vi "Hardware Discovery.vi"() -> ()   [LabVIEW 2020]
uses:
  support/Controls/State Data.ctl
  support/Controls/Targets Settings.ctl
  support/Controls/Target Information.ctl
  support/Controls/Target Network Settings.ctl
  support/Controls/System Credentials.ctl
  support/Controls/Important Paths.ctl
  support/Controls/Exit Button.ctl
  support/Controls/Refresh Button.ctl
  support/Controls/Configure Button.ctl
  support/Controls/Select All Button.ctl
  support/Controls/Add Target Button.ctl
  support/Controls/SetUp Btn.ctl
  support/Controls/FP Control Functions.ctl
  <vilib>/Utility/miscctls.llb/LVRowAndColumnUnsignedTypeDef.ctl
  support/Message Queue/Enqueue Message (Single).vi
  <vilib>/nisyscfg/Close (System).vi
  support/Message Queue/Message Queue.lvlib
  <vilib>/nisyscfg/nisyscfg.lvlib
  <resource>/objmgr/nisysapi.rc
  support/User Event - Stop/User Event - Stop.lvlib
panel:
  in  "App Images List":i32(listbox)=6
  in  "Target List 2":i32[](listbox)=[0]
  out "LinuxRT Version to be applied":string
  in  "Set Up Target":T1
  in  "Exit":T2
  in  "Target List":i32[](listbox)=[0]
  in  "Refresh Targets":T3
  in  "Targets Settings":bool
  in  "Add Target":T4
  in  "Select All":T5
  in  "Configure Targets":T6
  in  "App Data":T7 {"Targets Information"."Primary NIC"."IP Address Request Mode" items=["Static"=1, "DHCP/Link-Local"=2, "Link-Local Only"=4, "DHCP Only"=8]}
  # "Detected Targets"
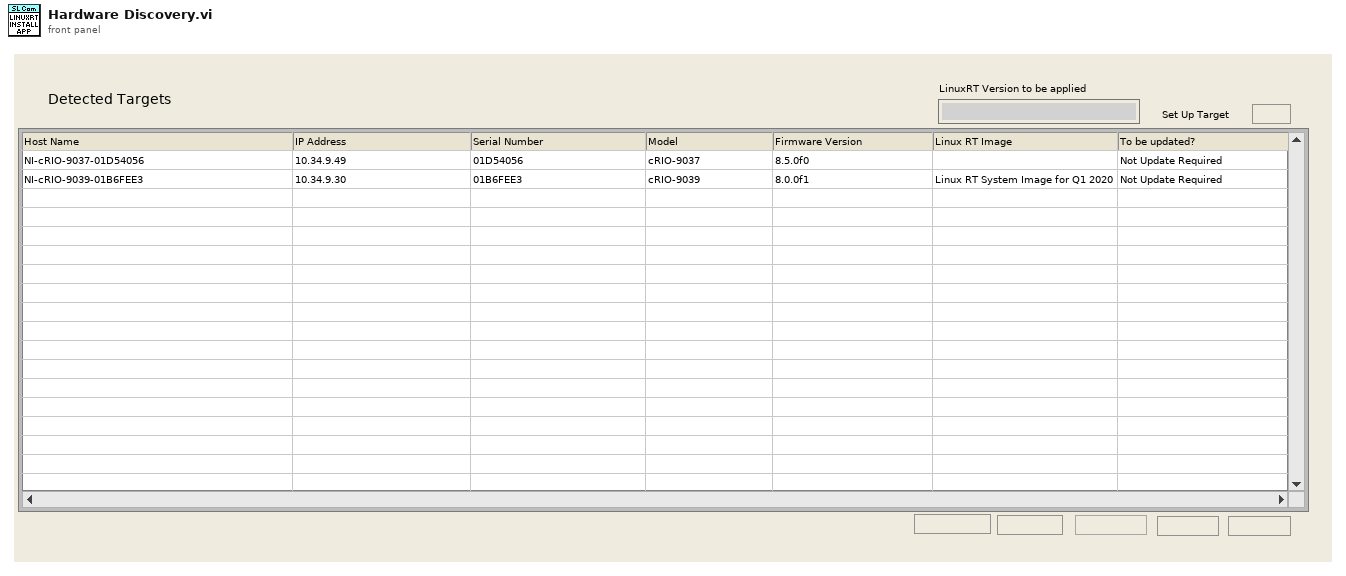
[diagram p1: front panel]
types:
  T1 = typedef "SetUp Btn.ctl" = bool
  T2 = typedef "Exit Button.ctl" = bool
  T3 = typedef "Refresh Button.ctl" = bool
  T4 = typedef "Add Target Button.ctl" = bool
  T5 = typedef "Select All Button.ctl" = bool
  T6 = typedef "Configure Button.ctl" = bool
  T7 = typedef "State Data.ctl" = cluster{"Targets Settings":T8, "Targets Information":T9[], "Filtered Targets":i32[], "User Added Targets":string[], "Important Paths":T12}
  T8 = typedef "Targets Settings.ctl" = cluster{"Target Types":string[], "Reduce Discovery Timeout":bool}
  T9 = typedef "Target Information.ctl" = cluster{"Hostname":string, "Serial number":string, "Product name":string, "Product code":i32, "System status":string, "Credential type":enum16{"None/Unlocked", "FTP Password", "NIAuth Credentials"}, "User added?":bool, "Primary NIC":T10, "System Credentials":T11}
  T10 = typedef "Target Network Settings.ctl" = cluster{"MAC address":string, "IP Address Request Mode":i32, "IP address":string, "Subnet mask":string, "Gateway":string, "DNS server":string}
  T11 = typedef "System Credentials.ctl" = cluster{"Username":string, "Password":string}
  T12 = typedef "Important Paths.ctl" = cluster{"System Configuration Version":string}
  T13 = typedef "LVPoint32TypeDef.ctl" = cluster{"Horizontal":i32, "Vertical":i32}
  T14 = typedef "LVRowAndColumnTypeDef.ctl" = cluster{"Row":i32, "Column":i32}
  T15 = typedef "LVRowAndColumnUnsignedTypeDef.ctl" = cluster{"Row":u32, "Column":u32}
  T16 = enum8{"Enabled", "Disabled", "Disabled and Grayed Out"}
  T17 = typedef "FP Control Functions.ctl" = enum16{"Open", "Close", "Bring To Front", "Center"}
  T18 = enum32{"invalid app kind", "Development System", "Run Time System", "Student Edition", "Embedded LabVIEW", "Evaluation", "Custom"}
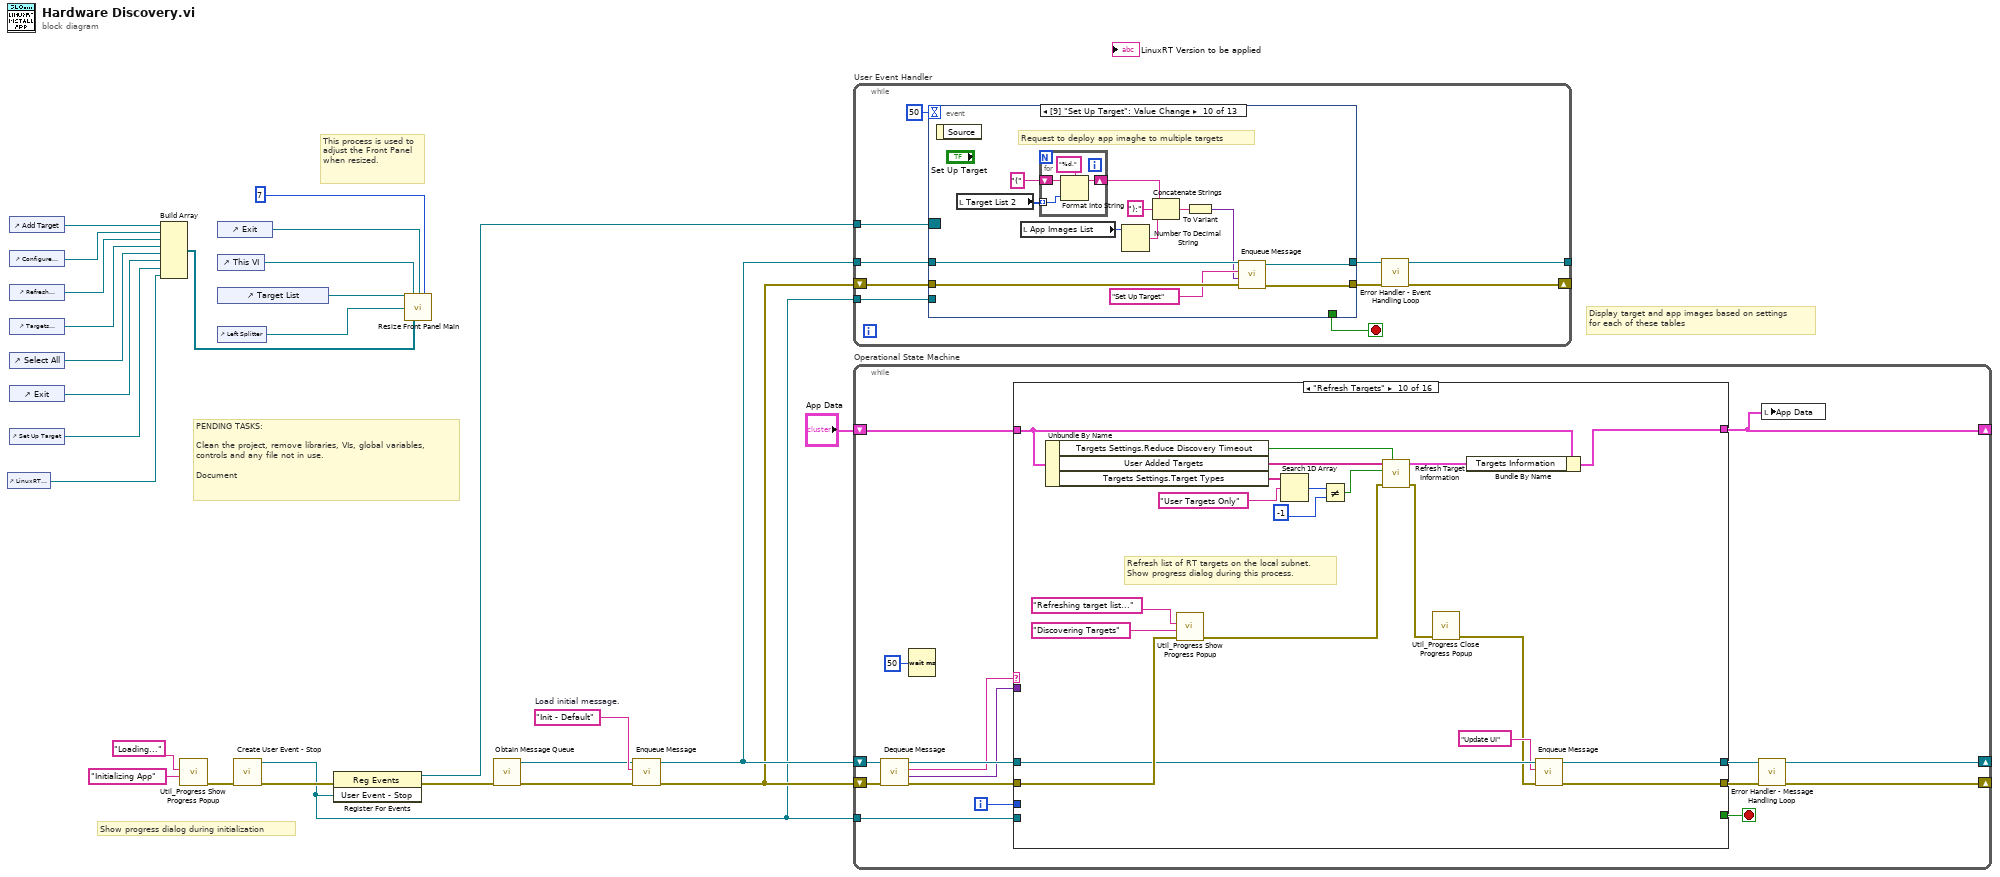
[diagram p0: block diagram]
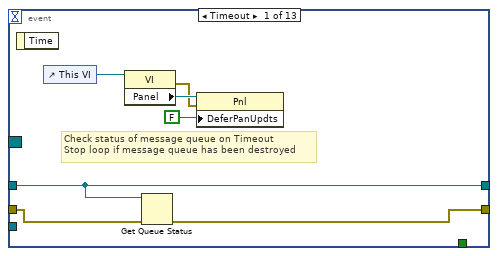
[diagram p2: hidden frame]
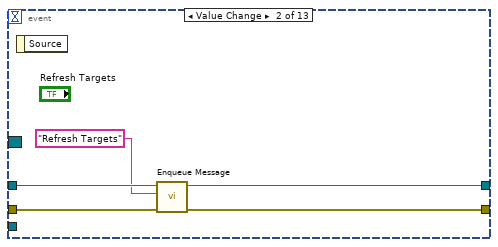
[diagram p3: hidden frame]
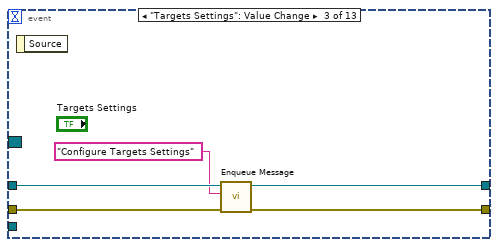
[diagram p4: hidden frame]
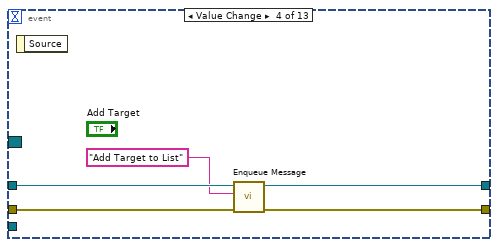
[diagram p5: hidden frame]
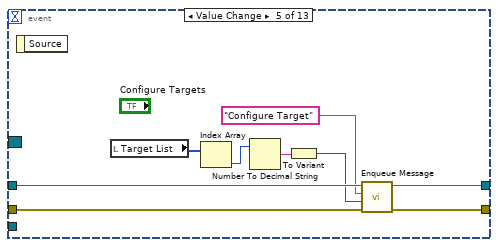
[diagram p6: hidden frame]
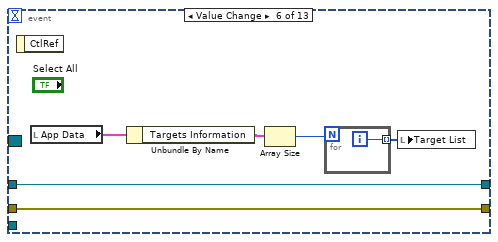
[diagram p7: hidden frame]
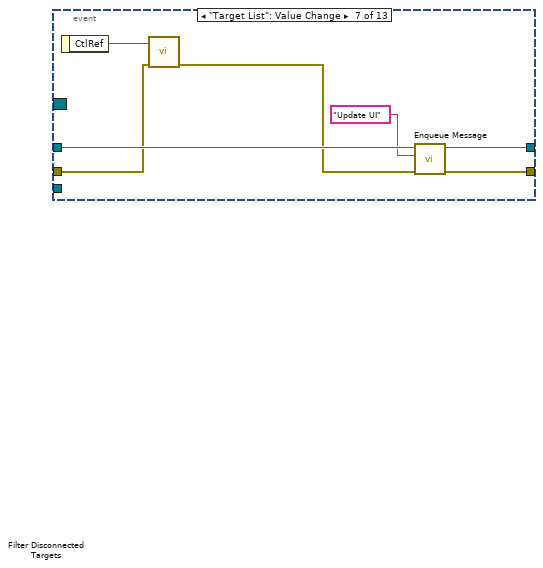
[diagram p8: hidden frame]
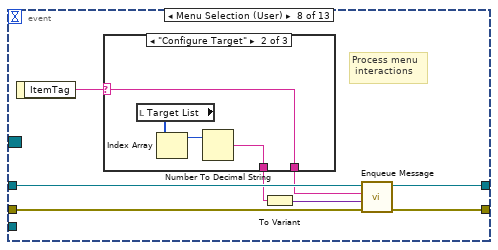
[diagram p9: hidden frame]
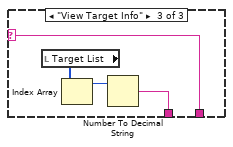
[diagram p11: hidden frame]
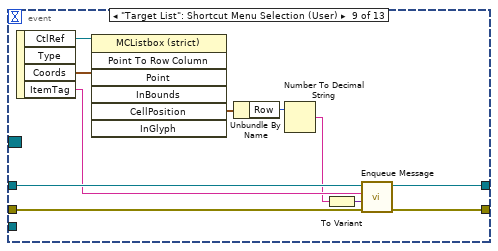
[diagram p12: hidden frame]
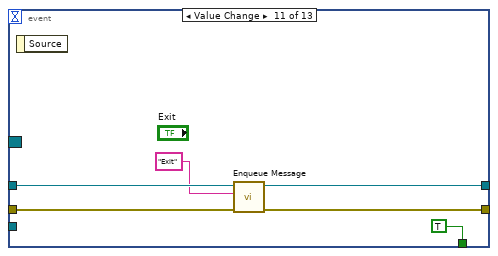
[diagram p13: hidden frame]
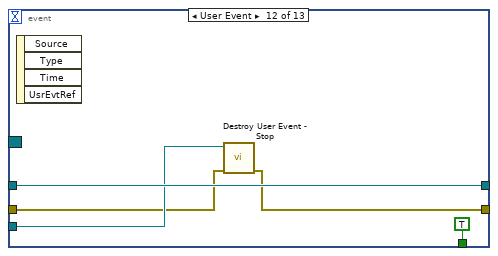
[diagram p14: hidden frame]
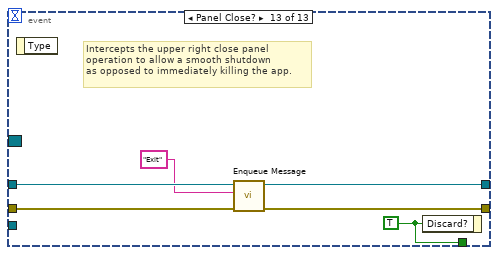
[diagram p15: hidden frame]
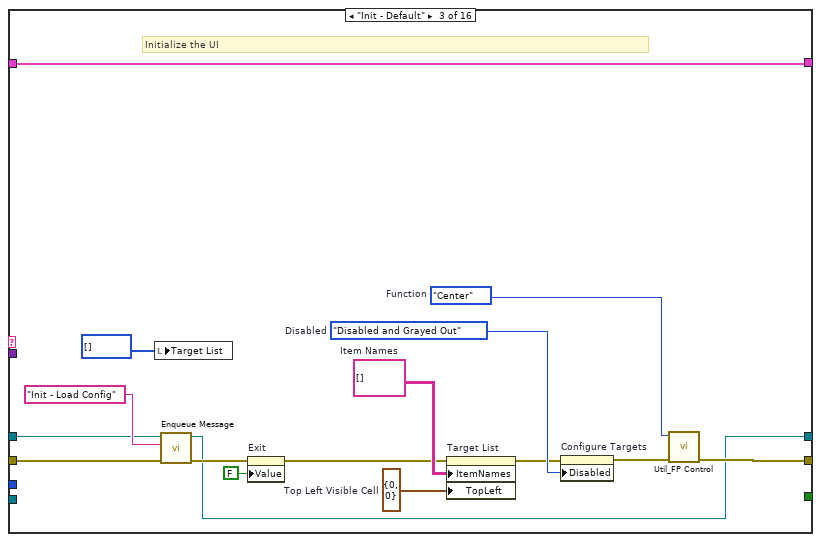
[diagram p18: hidden frame]
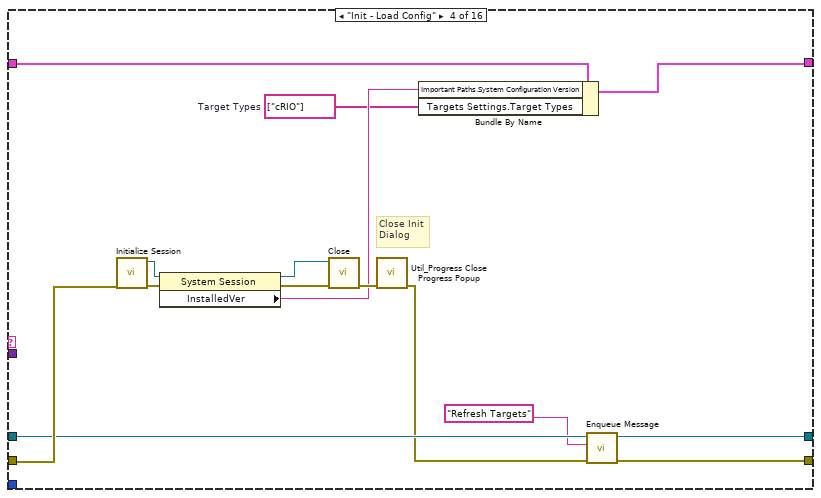
[diagram p19: hidden frame]
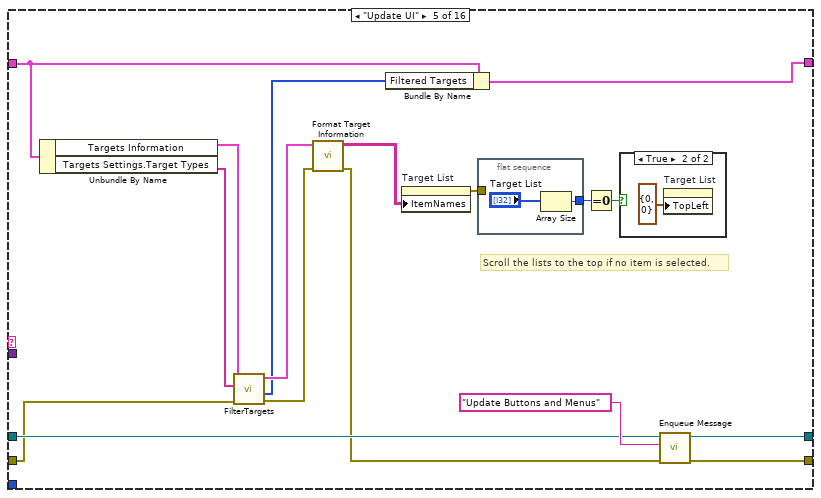
[diagram p20: hidden frame]
diagram:
  w15 = "Init - Default"  # Load initial message.
  # "PENDING TASKS:\n\nClean the project, remove libraries, VIs, global variables, \ncontrols and any file not in use.\n\nDocument"
  # "Display target and app images based on settings\nfor each of these tables"
  # "Show progress dialog during initialization"
  # "This process is used to adjust the Front Panel when resized."
  n1 = control-ref of="LinuxRT Version to be applied"() -> (w7:refnum<vi>)
  n2 = control-ref of="Add Target"() -> (w22:refnum<vi>)
  n3 = control-ref of="Configure Targets"() -> (w21:refnum<vi>)
  n4 = control-ref of="Refresh Targets"() -> (w20:refnum<vi>)
  n5 = control-ref of="Targets Settings"() -> (w19:refnum<vi>)
  n6 = control-ref of="Select All"() -> (w18:refnum<vi>)
  n7 = control-ref of="Exit"() -> (w11:refnum<vi>)
  n8 = control-ref of="Set Up Target"() -> (w8:refnum<vi>)
  n9 = Build Array(w22, w21, w20, w19, w18, w11, w8, w7) -> (w17:refnum<vi>[])
  n10 = call "Util_Progress Show Progress Popup.vi"("Title"="Initializing App", "Message"="Loading...") -> ("error out"=w5:errorcluster)  [unwired: 2 in, 7 out]
  n11 = control-ref of="Exit"() -> (w26:refnum<vi>)
  n12 = control-ref of="This VI"() -> (w25:refnum<vi>)
  n13 = control-ref of="Target List"() -> (w24:refnum<vi>)
  n14 = control-ref of="Left Splitter"() -> (w23:refnum<vi>)
  n15 = call "Create User Event - Stop.vi"("error in (no error)"=w5) -> ("error out"=w4:errorcluster, "User Event - Stop"=w1:refnum<user-event>)  [unwired: 9 in]
  n16 = register-events(error in=w4, w1) -> (reference out=w2:refnum<event-registration>, error out=w3:errorcluster)  [unwired: 1 in]
  n17 = call "Resize Front Panel Main.vi"("Left Listbox"=w24, "Top Level VI"=w25, "Stop"=w26, "Number of Columns"=7, "Left Splitter"=w23, "Left Pane Items"=w17) -> ()  [unwired: 9 in, 1 out]
  n18 = call "Obtain Message Queue.vi"("error in (no error)"=w3) -> ("error out"=w16:errorcluster, "Message Queue"=w14:refnum<queue>)  [unwired: 9 in]
  n19 = call-poly "Enqueue Message.vi"("error in (no error)"=w16, "Message"=w15, "Message Queue"=w14) -> ("error out"=w6:errorcluster, "dup Message Queue"=w13:refnum<queue>)  [unwired: 7 in]
  n20 = while "User Event Handler" {
    tunnel: w13 -> [w35]
    shift-right: [w31] -> _
    shift-left: w6 -> [w34]
    tunnel: w2 -> [w30]
    tunnel: w1 -> [w29]
    tunnel: [w28] -> _
    stop <- w36 stop-if-true
    n21 = event shown="[9] \"Set Up Target\": Value Change" {
      selector: w30 -> [_ _ _ _ _ _ _ _ _ _ _ _ _]
      dyn-events: _ -> [_ _ _ _ _ _ _ _ _ _ _ _ _]
      timeout: 50 -> [_ _ _ _ _ _ _ _ _ _ _ _ _]
      tunnel: [_ _ _ _ _ _ _ _ _ _ TRUE ("Discard?") TRUE ("Discard?") w144] -> w36
      tunnel: w35 -> [w44 w49 w52 w57 w64 w70 w80 w87 w104 w123 w130 w138 w141]
      tunnel: [w44 w48 w51 w56 w63 w70 w79 w86 w103 w121 w129 w138 w140] -> w32
      tunnel: w34 -> [w39 w47 w54 w59 w66 w69 w76 w89 w106 w122 w132 w135 w143]
      tunnel: [w38 w46 w53 w58 w65 w69 w81 w88 w105 w120 w131 w134 w142] -> w33
      tunnel: w29 -> [_ _ _ _ _ _ _ _ _ _ _ w136 _]
      event Timeout {
        # "Check status of message queue on Timeout\nStop loop if message queue has been destroyed"
        n22 = event-data() -> ()  [unwired: 2 out]
        n23 = control-ref of="This VI"() -> (w40:refnum<vi>)
        n24 = property class="VI"(reference=w40) -> (error out=w41:errorcluster, "Panel"=w43:refnum<vi>)  [unwired: 1 in, 1 out]
        n25 = Get Queue Status(queue=w44, error in (no error)=w39) -> (error out=w38:errorcluster)  [unwired: 8 out]
        n26 = property class="Pnl"(reference=w43, error in=w41, "DeferPanUpdts"=FALSE ("Defer Panel Updates")) -> ()  [unwired: 2 out]
      }
      event Value Change {
        n27 = event-data() -> ()  [unwired: 2 out]
        n28 = call-poly "Enqueue Message.vi"("error in (no error)"=w47, "Message"="Refresh Targets", "Message Queue"=w49) -> ("error out"=w46:errorcluster, "dup Message Queue"=w48:refnum<queue>)  [unwired: 7 in]
      }
      event "Targets Settings": Value Change {
        n29 = event-data() -> ()  [unwired: 2 out]
        n30 = call-poly "Enqueue Message.vi"("error in (no error)"=w54, "Message"="Configure Targets Settings", "Message Queue"=w52) -> ("error out"=w53:errorcluster, "dup Message Queue"=w51:refnum<queue>)  [unwired: 7 in]
      }
      event Value Change {
        n31 = event-data() -> ()  [unwired: 2 out]
        n32 = call-poly "Enqueue Message.vi"("error in (no error)"=w59, "Message"="Add Target to List" ("Message Name"), "Message Queue"=w57) -> ("error out"=w58:errorcluster, "dup Message Queue"=w56:refnum<queue>)  [unwired: 7 in]
      }
      event Value Change {
        n33 = event-data() -> ()  [unwired: 2 out]
        n34 = local read "Target List"() -> (w67:i32[])
        n35 = Index Array(array=w67) -> (element=w68:i32)  [unwired: 1 in]
        n36 = Number To Decimal String(number=w68) -> (decimal integer string=w62:string)  [unwired: 1 out]
        n37 = To Variant(anything=w62) -> (Variant=w61:variant)
        n38 = call-poly "Enqueue Message.vi"("error in (no error)"=w66, "Message Data"=w61, "Message"="Configure Target", "Message Queue"=w64) -> ("error out"=w65:errorcluster, "dup Message Queue"=w63:refnum<queue>)  [unwired: 6 in]
      }
      event Value Change {
        n39 = event-data() -> ()  [unwired: 2 out]
        n40 = local read "App Data"() -> (w73:T7)
        n41 = Unbundle By Name(w73) -> ("Targets Information"=w72:T9[])
        n42 = Array Size(array=w72) -> (size(s)=w71:i32)
        n43 = for {
          N: w71 -> [_]
          tunnel: [w75] -> w74 mode=indexing
          i -> [w75]
        }
        n44 = local write "Target List"(w74) -> ()
      }
      event "Target List": Value Change {
        n45 = event-data() -> ("CtlRef"=w82:refnum<vi>)  [unwired: 1 out]
        n46 = call "Filter Disconnected Targets.vi"("error in (no error)"=w76, "Target List Ref"=w82) -> ("error out"=w77:errorcluster)  [unwired: 9 in]
        n47 = call-poly "Enqueue Message.vi"("error in (no error)"=w77, "Message"="Update UI", "Message Queue"=w80) -> ("error out"=w81:errorcluster, "dup Message Queue"=w79:refnum<queue>)  [unwired: 7 in]
      }
      event Menu Selection (User) {
        # "Process menu\n interactions"
        n48 = event-data() -> ("ItemTag"=w90:string)  [unwired: 1 out]
        n49 = case shown="\"Configure Target\"" w90 {
          selector: w90 -> [w91 w93 w97]
          tunnel: [w91 w93 w97] -> w85
          tunnel: [_ w92 w96] -> w84
          frame Default {
          }
          frame "Configure Target" {
            n50 = local read "Target List"() -> (w95:i32[])
            n51 = Index Array(array=w95) -> (element=w94:i32)  [unwired: 1 in]
            n52 = Number To Decimal String(number=w94) -> (decimal integer string=w92:string)  [unwired: 1 out]
          }
          frame "View Target Info" {
            n53 = local read "Target List"() -> (w99:i32[])
            n54 = Index Array(array=w99) -> (element=w98:i32)  [unwired: 1 in]
            n55 = Number To Decimal String(number=w98) -> (decimal integer string=w96:string)  [unwired: 1 out]
          }
        }
        n56 = To Variant(anything=w84) -> (Variant=w83:variant)
        n57 = call-poly "Enqueue Message.vi"("error in (no error)"=w89, "Message Data"=w83, "Message"=w85, "Message Queue"=w87) -> ("error out"=w88:errorcluster, "dup Message Queue"=w86:refnum<queue>)  [unwired: 6 in]
      }
      event "Target List": Shortcut Menu Selection (User) {
        n58 = event-data() -> ("CtlRef"=w108:refnum<vi>, "Coords"=w107:T13, "ItemTag"=w102:string)  [unwired: 2 out]
        n59 = invoke class="MCListbox (strict)" method="Point To Row Column"(reference=w108, "Point"=w107) -> ("CellPosition"=w110:T14)  [unwired: 5 in, 6 out]
        n60 = Unbundle By Name(w110) -> ("Row"=w109:i32)
        n61 = Number To Decimal String(number=w109) -> (decimal integer string=w101:string)  [unwired: 1 out]
        n62 = To Variant(anything=w101) -> (Variant=w100:variant)
        n63 = call-poly "Enqueue Message.vi"("error in (no error)"=w106, "Message Data"=w100, "Message"=w102, "Message Queue"=w104) -> ("error out"=w105:errorcluster, "dup Message Queue"=w103:refnum<queue>)  [unwired: 6 in]
      }
      event Value Change {
        # "Request to deploy app imaghe to multiple targets"
        n64 = event-data() -> ()  [unwired: 2 out]
        n65 = local read "Target List 2"() -> (w117:i32[])
        n66 = local read "App Images List"() -> (w115:i32)
        n67 = for {
          shift-right: [w127] -> w118
          shift-left: "(" -> [w125]
          tunnel: w117 -> [w126] mode=indexing
          n68 = Format Into String(format string="%d,", initial string=w125, w126) -> (resulting string=w127:string)  [unwired: 1 in, 1 out]
        }
        n69 = Number To Decimal String(number=w115) -> (decimal integer string=w114:string)  [unwired: 1 out]
        n70 = Concatenate Strings(w118, "):" ("string"), w114) -> (w112:string)
        n71 = To Variant(anything=w112) -> (Variant=w111:variant)
        n72 = call-poly "Enqueue Message.vi"("error in (no error)"=w122, "Message Data"=w111, "Message"="Set Up Target", "Message Queue"=w123) -> ("error out"=w120:errorcluster, "dup Message Queue"=w121:refnum<queue>)  [unwired: 6 in]
      }
      event Value Change {
        n73 = event-data() -> ()  [unwired: 2 out]
        n74 = call-poly "Enqueue Message.vi"("error in (no error)"=w132, "Message"="Exit", "Message Queue"=w130) -> ("error out"=w131:errorcluster, "dup Message Queue"=w129:refnum<queue>)  [unwired: 7 in]
      }
      event User Event {
        n75 = event-data() -> ()  [unwired: 5 out]
        n76 = call "Destroy User Event - Stop.vi"("error in (no error)"=w135, "User Event - Stop"=w136) -> ("error out"=w134:errorcluster)  [unwired: 9 in]
      }
      event Panel Close? {
        w144 = TRUE ("Discard?")
        # "Intercepts the upper right close panel\noperation to allow a smooth shutdown\nas opposed to immediately killing the app."
        n77 = event-data() -> ()  [unwired: 2 out]
        n78 = call-poly "Enqueue Message.vi"("error in (no error)"=w143, "Message"="Exit", "Message Queue"=w141) -> ("error out"=w142:errorcluster, "dup Message Queue"=w140:refnum<queue>)  [unwired: 7 in]
        n79 = event-data("Discard?"=w144) -> ()  [unwired: 1 in, 1 out]
      }
    }
    n80 = call "Error Handler - Event Handling Loop.vi"("error in (no error)"=w33, "Message Queue"=w32) -> ("dup error in"=w31:errorcluster, "dup Message Queue"=w28:refnum<queue>)  [unwired: 8 in]
  }
  n81 = while "Operational State Machine" {
    shift-left: w6 -> [w158]
    shift-right: [w149] -> _
    shift-right: [w152] -> _
    shift-left: "App Data" -> [w153]
    shift-right: [w147] -> _
    shift-left: w13 -> [w156]
    tunnel: w1 -> [w146]
    i -> [w160]
    stop <- w151 stop-if-true
    n82 = call "Dequeue Message.vi"("error in (no error)"=w158, "Message Queue"=w156) -> ("error out"=w157:errorcluster, "Message Data"=w154:variant, "Message"=w145:string, "dup Message Queue"=w155:refnum<queue>)  [unwired: 6 in]
    n83 = Wait (ms)(milliseconds to wait=u32 50) -> ()  [unwired: 1 out]
    n84 = case shown="\"Refresh Targets\"" w145 {
      tunnel: [w162 w165 w167 w188 w205 w226 w228 w242 w255 w260 w279 w308 w323 w343 w357 w372] -> w152
      tunnel: w155 -> [w161 w164 w176 w190 w202 w218 w227 w232 w254 w262 w282 w310 w329 w338 w355 w369]
      tunnel: w157 -> [w163 w166 w178 w192 w198 w219 w230 w241 w256 w268 w284 w306 w328 w346 w356 w362]
      tunnel: w160 -> [_ _ _ _ _ _ _ _ _ _ _ _ _ _ _ _]
      tunnel: w154 -> [_ _ _ _ _ _ _ _ _ _ _ w307 _ w341 _ w366]
      tunnel: [w163 w166 w173 w193 w204 w220 errorcluster {"status"=FALSE, "code"=0, "source"=""} ("error out") w237 w256 w263 w283 w312 w325 w337 w356 w370] -> w150
      tunnel: w153 -> [w162 w165 w167 w186 w206 w226 w228 w242 w255 w259 w280 w309 w321 w343 w357 w372]
      tunnel: [_ _ _ _ _ _ _ TRUE _ _ _ _ _ _ _ _] -> w151
      tunnel: [w161 w164 w168 w183 w200 w218 w227 w232 w254 w257 w277 w302 w322 w338 w355 w368] -> w148
      tunnel: w146 -> [_ _ _ _ _ _ _ w234 _ _ _ _ _ _ _ _]
      frame "Missing Message Handler", Default {
      }
      frame "**** General Application Messages ****" {
      }
      frame "Init - Default" {
        w175 = T16."Disabled and Grayed Out"  # Disabled
        w179 = T15 {"Row"=0, "Column"=0}  # Top Left Visible Cell
        w180 = FP_Control_Functions."Center"  # Function
        w181 = string[][] []  # Item Names
        # "Initialize the UI"
        n85 = local write "Target List"(i32[] [] ("Target List")) -> ()
        n86 = call-poly "Enqueue Message.vi"("error in (no error)"=w178, "Message"="Init - Load Config", "Message Queue"=w176) -> ("error out"=w171:errorcluster, "dup Message Queue"=w168:refnum<queue>)  [unwired: 7 in]
        n87 = property on="Exit" class="Bool (strict)"(error in=w171, "Value"=T2 FALSE ("Exit")) -> (error out=w170:errorcluster)  [unwired: 1 in, 1 out]
        n88 = property on="Target List" class="MCListbox (strict)"(error in=w170, "ItemNames"=w181, "TopLeft"=w179) -> (error out=w174:errorcluster)  [unwired: 1 in, 1 out]
        n89 = property on="Configure Targets" class="Bool"(error in=w174, "Disabled"=w175) -> (error out=w172:errorcluster)  [unwired: 1 in, 1 out]
        n90 = call "Util_FP Control.vi"("error in (no error)"=w172, "Function"=w180) -> ("error out"=w173:errorcluster)  [unwired: 9 in]
      }
      frame "Init - Load Config" {
        w184 = string[] ["cRIO"]  # Target Types
        # "Close Init\nDialog"
        n91 = call <vilib>:"Initialize Session.vi"("error in (no error)"=w192) -> ("error out"=w195:errorcluster, "Session out"=w196:refnum<k21>)  [unwired: 9 in]
        n92 = property class="System Session"(reference=w196, error in=w195) -> (reference out=w197:refnum<k21>, error out=w194:errorcluster, "InstalledVer"=w187:string)
        n93 = call-poly <vilib>:"Close.vi"("error in (no error)"=w194, "Session in"=w197) -> ("error out"=w191:errorcluster)  [unwired: 9 in]
        n94 = call "Util_Progress Close Progress Popup.vi"("error in (no error)"=w191) -> ("error out"=w189:errorcluster)  [unwired: 2 in, 8 out]
        n95 = Bundle By Name(cluster=w186, "Important Paths.System Configuration Version"=w187, "Targets Settings.Target Types"=w184) -> (w188:T7)
        n96 = call-poly "Enqueue Message.vi"("error in (no error)"=w189, "Message"="Refresh Targets", "Message Queue"=w190) -> ("error out"=w193:errorcluster, "dup Message Queue"=w183:refnum<queue>)  [unwired: 7 in]
      }
      frame "Update UI" {
        # "Scroll the lists to the top if no item is selected."
        n97 = Unbundle By Name(w206) -> ("Targets Information"=w214:T9[], "Targets Settings.Target Types"=w210:string[])
        n98 = call "FilterTargets.vi"("error in (no error)"=w198, "Target Types"=w210, "Targets Information"=w214) -> ("error out"=w201:errorcluster, "Filtered Targets"=w212:i32[], "Targets Information"=w213:T9[])  [unwired: 6 out]
        n99 = call "Format Target Information.vi"("error in"=w201, "Targets Information"=w213) -> ("error out"=w199:errorcluster, "Targets Information"=w211:string[][])  [unwired: 8 out]
        n100 = Bundle By Name(cluster=w206, "Filtered Targets"=w212) -> (w205:T7)
        n101 = property on="Target List" class="MCListbox (strict)"("ItemNames"=w211) -> (error out=w209:errorcluster)  [unwired: 2 in, 1 out]
        n102 = flat-sequence {
          tunnel: w209 -> [_]
          tunnel: [w216] -> w208
          frame #0 {
            n103 = Array Size(array="Target List") -> (size(s)=w216:i32)
          }
        }
        n104 = Equal To 0?(x=w208) -> (x = 0?=w207:bool)
        n105 = case shown="True" w207 {
          frame False {
          }
          frame True {
            n106 = property on="Target List" class="MCListbox (strict)"("TopLeft"=T15 {"Row"=0, "Column"=0} ("Top Left Visible Cell")) -> ()  [unwired: 2 in, 2 out]
          }
        }
        n107 = call-poly "Enqueue Message.vi"("error in (no error)"=w199, "Message"="Update Buttons and Menus" ("Message Name"), "Message Queue"=w202) -> ("error out"=w204:errorcluster, "dup Message Queue"=w200:refnum<queue>)  [unwired: 7 in]
      }
      frame "Update Buttons and Menus" {
        n108 = local read "Target List"() -> (w225:i32[])
        n109 = call "Button and Menu Status.vi"("Target List"=w225) -> ("Configure Target"=w222:bool)  [unwired: 9 in, 1 out]
        n110 = Select(t=T16."Enabled" ("Disabled"), s=w222, f=T16."Disabled and Grayed Out" ("Disabled")) -> (s? t:f=w221:T16)
        n111 = property on="Configure Targets" class="Bool"(error in=w219, "DisabledEnum"=w221) -> (error out=w220:errorcluster)  [unwired: 1 in, 1 out]
      }
      frame "Error" {
        # "Display run-time error message\nAdd code to log error if desired"
        n112 = disable-structure shown="TARGET_TYPE==Windows" {
          disable-tunnel: w230 -> [w231 _]
          frame condition #0 (active) {
            n113 = call <vilib>:"Simple Error Handler.vi"("error in (no error)"=w231) -> ()  [unwired: 1 in, 8 out]
          }
          frame condition #1 {
          }
        }
      }
      frame "Exit" {
        # "Close the front panel if the application is running as an EXE"
        n114 = call <vilib>:"Clear Errors.vi"("error in (no error)"=w241) -> ("error out"=w233:errorcluster)  [unwired: 5 in, 1 out]
        n115 = Open Application Reference(8:w241) -> (0:w244:errorcluster, 3:w245:refnum<vi>)  [unwired: 3 in]
        n116 = property class="App"(reference=w245, error in=w244) -> (error out=w240:errorcluster, "App.Kind"=w243:T18)  [unwired: 1 out]
        n117 = call "Fire User Event - Stop.vi"("error in (no error)"=w233, "User Event - Stop"=w234) -> ("error out"=w236:errorcluster)  [unwired: 9 in]
        n118 = case shown="Default" w243 {
          tunnel: w240 -> [w248 w250]
          tunnel: [w248 w249] -> w239
          frame Default {
          }
          frame "Run Time System" {
            # "Close FP in EXE"
            n119 = Current VI's Path() -> (path=w253:path)
            n120 = Open VI Reference(vi path=w253, error in (no error)=w250) -> (vi reference=w252:refnum<vi>, error out=w251:errorcluster)  [unwired: 4 in]
            n121 = invoke class="VI" method="FP.Close"(reference=w252, error in=w251) -> (error out=w249:errorcluster)  [unwired: 1 in, 2 out]
          }
        }
        n122 = Merge Errors(w239, w236) -> (w238:errorcluster)
        n123 = flat-sequence {
          tunnel: w238 -> [w247]
          tunnel: [w247] -> w237
          frame #0 {
            n124 = local write "Exit"(T2 FALSE ("Exit")) -> ()
          }
        }
      }
      frame "**** Target Messages ****" {
      }
      frame "Refresh Targets" {
        # "Refresh list of RT targets on the local subnet.\nShow progress dialog during this process."
        n125 = Unbundle By Name(w259) -> ("Targets Settings.Reduce Discovery Timeout"=w266:bool, "User Added Targets"=w274:string[], "Targets Settings.Target Types"=w265:string[])
        n126 = call "Util_Progress Show Progress Popup.vi"("error in (no error)"=w268, "Title"="Discovering Targets", "Message"="Refreshing target list...") -> ("error out"=w267:errorcluster)  [unwired: 1 in, 7 out]
        n127 = Search 1D Array(1D array=w265, element="User Targets Only") -> (index of element=w271:i32)  [unwired: 1 in]
        n128 = Not Equal?(x=w271, y=-1) -> (x != y?=w269:bool)
        n129 = call "Refresh Target Information.vi"("Reduce Discovery Timeout"=w266, "error in (no error)"=w267, "User Added Targets Only"=w269, "User Added Targets"=w274) -> ("error out"=w264:errorcluster, "Targets Information"=w273:T9[])  [unwired: 6 in]
        n130 = call "Util_Progress Close Progress Popup.vi"("error in (no error)"=w264) -> ("error out"=w258:errorcluster)  [unwired: 2 in, 8 out]
        n131 = Bundle By Name(cluster=w259, "Targets Information"=w273) -> (w260:T7)
        n132 = call-poly "Enqueue Message.vi"("error in (no error)"=w258, "Message"="Update UI", "Message Queue"=w262) -> ("error out"=w263:errorcluster, "dup Message Queue"=w257:refnum<queue>)  [unwired: 7 in]
      }
      frame "Add Target to List" {
        n133 = Unbundle By Name(w280) -> ("User Added Targets"=w286:string[])
        n134 = call "Add Target By IP Dialog.vi"() -> ("Canceled?"=w281:bool, "IP Address"=w285:string)  [unwired: 10 in]
        n135 = case shown="False" w281 {
          tunnel: w286 -> [w296 w301]
          tunnel: w285 -> [w295 _]
          tunnel: [w297 w301] -> w278
          frame False {
            n136 = Search 1D Array(1D array=w296, element=w295) -> (index of element=w300:i32)  [unwired: 1 in]
            n137 = Build Array (concatenate)(w296, w295) -> (w294:string[])
            n138 = Not Equal?(x=w300, y=-1) -> (x != y?=w298:bool)
            n139 = Select(t=w296, s=w298, f=w294) -> (s? t:f=w297:string[])
          }
          frame True {
          }
        }
        n140 = case shown="False" w281 {
          tunnel: w284 -> [w291 w293]
          tunnel: [w290 w293] -> w283
          tunnel: w282 -> [w288 w292]
          tunnel: [w287 w292] -> w277
          frame False {
            n141 = call-poly "Enqueue Message.vi"("error in (no error)"=w291, "Message"="Refresh Targets" ("Message Name"), "Message Queue"=w288) -> ("error out"=w290:errorcluster, "dup Message Queue"=w287:refnum<queue>)  [unwired: 7 in]
          }
          frame True {
          }
        }
        n142 = Bundle By Name(cluster=w280, "User Added Targets"=w278) -> (w279:T7)
      }
      frame "Configure Target" {
        # "Update network settings/configuration of the selected RT target"
        n143 = Variant To Data(error in=w306, type="", Variant=w307) -> (data=w303:string, error out=w305:errorcluster)
        n144 = Unbundle By Name(w309) -> ("Targets Information"=w317:T9[], "Filtered Targets"=w320:i32[])
        n145 = Decimal String To Number(string=w303) -> (number=w319:i32)  [unwired: 3 out]
        n146 = Index Array(array=w320, index=w319) -> (element=w315:i32)
        n147 = Index Array(array=w317, index=w315) -> (element=w318:T9)
        n148 = call "Configure Target Dialog.vi"("Error In"=w305, "Target Information in"=w318) -> ("Error Out"=w313:errorcluster, "Target Information out"=w316:T9)  [unwired: 8 out]
        n149 = Replace Array Subset(array=w317, new element=w316, index=w315) -> (w314:T9[])
        n150 = call <vilib>:"General Error Handler.vi"("error in (no error)"=w313) -> ()  [unwired: 10 in, 5 out]
        n151 = Bundle By Name(cluster=w309, "Targets Information"=w314) -> (w308:T7)
        n152 = call-poly "Enqueue Message.vi"("error in (no error)"=w305, "Message"="Update UI", "Message Queue"=w310) -> ("error out"=w312:errorcluster, "dup Message Queue"=w302:refnum<queue>)  [unwired: 7 in]
      }
      frame "Configure Targets Settings" {
        # "Configures the Global Timeout"
        n153 = Unbundle By Name(w321) -> ("Targets Settings"=w326:T8)
        n154 = call "Configure Targets Settings Dialog.vi"("Targets Settings"=w326) -> ("Targets Settings"=w327:T8)  [unwired: 10 out]
        n155 = Equal?(x=w327, y=w326) -> (x = y?=w324:bool)
        n156 = Bundle By Name(cluster=w321, "Targets Settings"=w327) -> (w323:T7)
        n157 = case shown="False" w324 {
          tunnel: w329 -> [w332 w335]
          tunnel: w328 -> [w334 w336]
          tunnel: [w333 w336] -> w325
          tunnel: [w330 w335] -> w322
          frame False {
            n158 = call-poly "Enqueue Message.vi"("error in (no error)"=w334, "Message"="Update UI", "Message Queue"=w332) -> ("error out"=w333:errorcluster, "dup Message Queue"=w330:refnum<queue>)  [unwired: 7 in]
          }
          frame True {
          }
        }
      }
      frame "View Target Info" {
        # "Display additional information about \nthe selected RT target in a popup window"
        n159 = Variant To Data(error in=w346, type="", Variant=w341) -> (data=w340:string, error out=w342:errorcluster)
        n160 = Unbundle By Name(w343) -> ("Targets Information"=w351:T9[], "Filtered Targets"=w350:i32[])
        n161 = Decimal String To Number(string=w340) -> (number=w349:i32)  [unwired: 3 out]
        n162 = Index Array(array=w350, index=w349) -> (element=w348:i32)
        n163 = Index Array(array=w351, index=w348) -> (element=w344:T9)
        n164 = call "Get Target Info (IP).vi"("error in (no error)"=w342, "Target settings in"=w344) -> ("error out"=w345:errorcluster, "Target settings out"=w347:T9)  [unwired: 8 in]
        n165 = case shown="No Error" w345 {
          selector: w345 -> [w352 w354]
          tunnel: w347 -> [w353 _]
          tunnel: [w352 w354] -> w337
          frame No Error {
            n166 = call "Target Info Dialog.vi"("Target Information"=w353) -> ()  [unwired: 11 out]
          }
          frame Error {
          }
        }
      }
      frame "*** SW Installation Message ****" {
      }
      frame "Set Up Target" {
        # "Filters selected targets"
        n167 = Variant To Data(error in=w362, type="", Variant=w366) -> (data=w360:string)  [unwired: 1 out]
        n168 = Unbundle By Name(w372) -> ("Targets Information"=w364:T9[], "Filtered Targets"=w365:i32[])
        n169 = Scan From String(format string="(%[^)]):%d", input string=w360) -> (output 1=w359:string)  [unwired: 2 in, 6 out]
        n170 = while {
          shift-right: [w379] -> _
          shift-left: w359 -> [w381]
          tunnel: w365 -> [w376]
          tunnel: w364 -> [w374]
          tunnel: [w373] -> w358 mode=indexing
          stop <- w378 stop-if-true
          n171 = Scan From String(format string="%d,", input string=w381) -> (remaining string=w379:string, output 1=w375:i32)  [unwired: 2 in, 3 out]
          n172 = Index Array(array=w376, index=w375) -> (element=w377:i32)
          n173 = Empty String/Path?(string/path=w379) -> (empty?=w378:bool)
          n174 = Index Array(array=w374, index=w377) -> (element=w373:T9)
        }
        n175 = call "Install Linux Image.vi"("error in (no error)"=w362, "Selected Targets"=w358) -> ("error out"=w371:errorcluster)  [unwired: 8 in, 1 out]
        n176 = call-poly "Enqueue Message.vi"("error in (no error)"=w371, "Message"="Refresh Targets", "Message Queue"=w369) -> ("error out"=w370:errorcluster, "dup Message Queue"=w368:refnum<queue>)  [unwired: 7 in]
      }
    }
    n177 = call "Error Handler - Message Handling Loop.vi"("error in (no error)"=w150, "Message Queue"=w148) -> ("dup error in"=w149:errorcluster, "dup Message Queue"=w147:refnum<queue>)  [unwired: 8 in]
    n178 = local write "App Data"(w152) -> ()
  }
